vi "Button Decode To String.vi"(11 "button info":T1) -> (3 "decoded button string":string)   [LabVIEW 2014, in "Joystick Fight Simulator.lvlib"]
doc: "Buttons are at input in cluster, here unbundle them, make array from them, convert it into number and then provide string based on that number, to get some human readible string output."
uses:
  Joystick Fight Simulator.lvlib
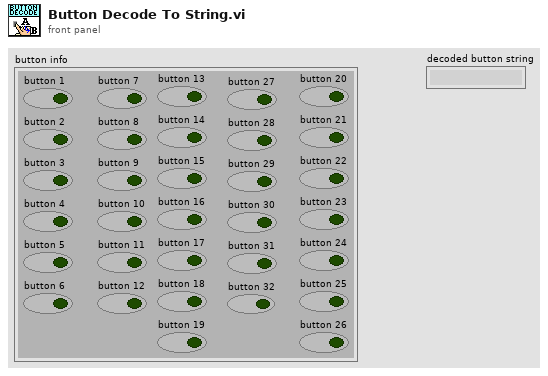
[diagram p1: front panel]
types:
  T1 = cluster{"button 1":bool, "button 2":bool, "button 3":bool, "button 4":bool, "button 5":bool, "button 6":bool, "button 7":bool, "button 8":bool, "button 9":bool, "button 10":bool, "button 11":bool, "button 12":bool, "button 13":bool, "button 14":bool, "button 15":bool, "button 16":bool, "button 17":bool, "button 18":bool, "button 19":bool, "button 20":bool, "button 21":bool, "button 22":bool, "button 23":bool, "button 24":bool, "button 25":bool, "button 26":bool, "button 32":bool, "button 31":bool, "button 30":bool, "button 29":bool, "button 28":bool, "button 27":bool}
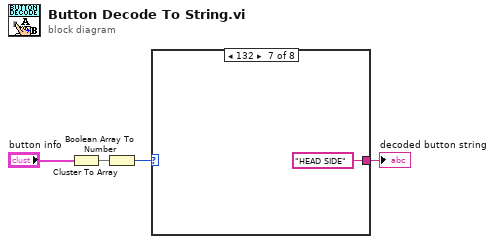
[diagram p0: block diagram]
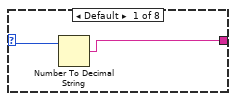
[diagram p2: hidden frame]
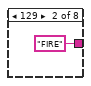
[diagram p3: hidden frame]
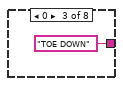
[diagram p4: hidden frame]
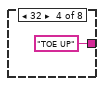
[diagram p5: hidden frame]
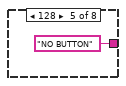
[diagram p6: hidden frame]
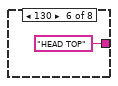
[diagram p7: hidden frame]
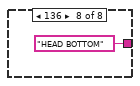
[diagram p8: hidden frame]
diagram:
  n1 = Cluster To Array(cluster="button info") -> (array=w4:bool[])
  n2 = Boolean Array To Number(Boolean array=w4) -> (number=w2:u32)
  n3 = case shown="132" w2 {
    selector: w2 -> [w6 _ _ _ _ _ _ _]
    tunnel: [w5 "FIRE" "TOE DOWN" "TOE UP" "NO BUTTON" "HEAD TOP" "HEAD SIDE" "HEAD BOTTOM"] -> w1
    frame Default {
      n4 = Number To Decimal String(number=w6) -> (decimal integer string=w5:string)  [unwired: 1 in]
    }
    frame 129 {
    }
    frame 0 {
    }
    frame 32 {
    }
    frame 128 {
    }
    frame 130 {
    }
    frame 132 {
    }
    frame 136 {
    }
  }
  "decoded button string" <- w1
